vi "publish status.vi"(8 "error in (no error)":errorcluster, 11 "Channel in":refnum<class "SPARC4_Channel.lvclass">) -> (0 "error out":errorcluster, 3 "Channel out":refnum<class "SPARC4_Channel.lvclass">)   [LabVIEW 2018, in "SPARC4_Channel.lvclass"]
uses:
  SPARC4_Channel.lvclass
  State Machine/State Machine.lvclass
  Sim_Ixon_Ultra/Sim_Ixon_Ultra.lvclass
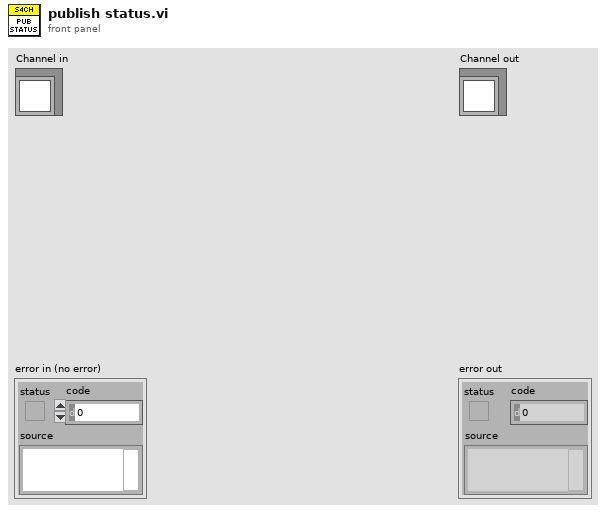
[diagram p1: front panel]
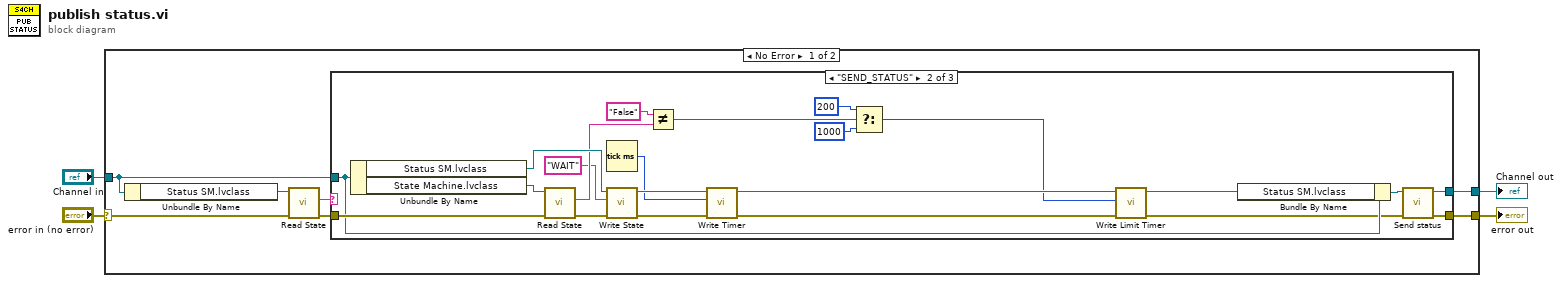
[diagram p0: block diagram]
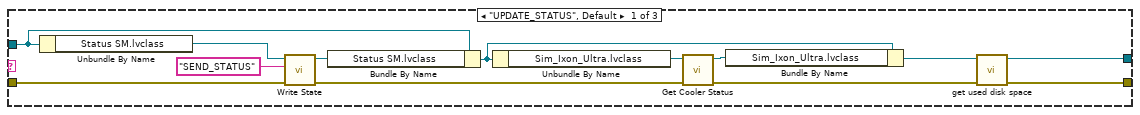
[diagram p2: hidden frame]
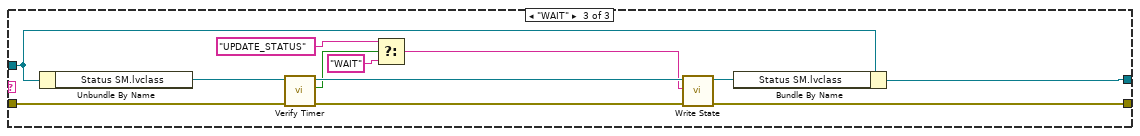
[diagram p3: hidden frame]
diagram:
  n1 = case shown="No Error" "error in (no error)" {
    selector: "error in (no error)" -> [w10 w60]
    tunnel: [w5 w60] -> w3
    tunnel: [w7 w59] -> w1
    tunnel: "Channel in" -> [w6 w59]
    frame No Error {
      n2 = Unbundle By Name(w6) -> ("Status SM.lvclass"=w11:refnum<class "State Machine.lvclass">)
      n3 = call-dynamic "Read State.vi"("error in (no error)"=w10, "State Machine in"=w11) -> ("error out"=w8:errorcluster, "State"=w9:string)  [unwired: 7 in, 1 out]
      n4 = case shown="\"SEND_STATUS\"" w9 {
        tunnel: w6 -> [w19 w30 w57]
        tunnel: w8 -> [w20 w31 w58]
        tunnel: [w14 w26 w51] -> w5
        tunnel: [w12 w25 w55] -> w7
        frame "UPDATE_STATUS", Default {
          n5 = Unbundle By Name(w19) -> ("Status SM.lvclass"=w22:refnum<class "State Machine.lvclass">)
          n6 = call-dynamic "Write State.vi"("error in (no error)"=w20, "State"="SEND_STATUS", "State Machine in"=w22) -> ("error out"=w17:errorcluster, "State Machine out"=w23:refnum<class "State Machine.lvclass">)  [unwired: 7 in]
          n7 = Bundle By Name(cluster=w19, "Status SM.lvclass"=w23) -> (w24:refnum<class "SPARC4_Channel.lvclass">)
          n8 = Unbundle By Name(w24) -> ("Sim_Ixon_Ultra.lvclass"=w18:refnum<class "Sim_Ixon_Ultra.lvclass">)
          n9 = call-dynamic "Get Cooler Status.vi"("error in (no error)"=w17, "CCDCamera in"=w18) -> ("error out"=w15:errorcluster, "CCDCamera out"=w16:refnum<class "Sim_Ixon_Ultra.lvclass">)  [unwired: 8 in]
          n10 = Bundle By Name(cluster=w24, "Sim_Ixon_Ultra.lvclass"=w16) -> (w13:refnum<class "SPARC4_Channel.lvclass">)
          n11 = call "get used disk space.vi"("error in (no error)"=w15, "Channel in"=w13) -> ("error out"=w14:errorcluster, "Channel out"=w12:refnum<class "SPARC4_Channel.lvclass">)  [unwired: 8 in]
        }
        frame "SEND_STATUS" {
          n12 = Unbundle By Name(w30) -> ("Status SM.lvclass"=w39:refnum<class "State Machine.lvclass">, "State Machine.lvclass"=w40:refnum<class "State Machine.lvclass">)
          n13 = call-dynamic "Read State.vi"("error in (no error)"=w31, "State Machine in"=w40) -> ("error out"=w38:errorcluster, "State"=w37:string)  [unwired: 7 in, 1 out]
          n14 = Tick Count (ms)() -> (millisecond timer value=w44:u32)
          n15 = call-dynamic "Write State.vi"("error in (no error)"=w38, "State"="WAIT", "State Machine in"=w39) -> ("error out"=w45:errorcluster, "State Machine out"=w46:refnum<class "State Machine.lvclass">)  [unwired: 7 in]
          n16 = Not Equal?(x="False" ("State"), y=w37) -> (x != y?=w29:bool)
          n17 = call "Write Timer.vi"("error in (no error)"=w45, "Timer"=w44, "State Machine in"=w46) -> ("error out"=w41:errorcluster, "State Machine out"=w43:refnum<class "State Machine.lvclass">)  [unwired: 7 in]
          n18 = Select(t=200, s=w29, f=1000) -> (s? t:f=w36:i32)
          n19 = call "Write Limit Timer.vi"("error in (no error)"=w41, "Limit Timer"=w36, "State Machine in"=w43) -> ("error out"=w27:errorcluster, "State Machine out"=w42:refnum<class "State Machine.lvclass">)  [unwired: 7 in]
          n20 = Bundle By Name(cluster=w30, "Status SM.lvclass"=w42) -> (w28:refnum<class "SPARC4_Channel.lvclass">)
          n21 = call "Send status.vi"("error in (no error)"=w27, "Channel in"=w28) -> ("error out"=w26:errorcluster, "Channel out"=w25:refnum<class "SPARC4_Channel.lvclass">)  [unwired: 8 in]
        }
        frame "WAIT" {
          n22 = Unbundle By Name(w57) -> ("Status SM.lvclass"=w56:refnum<class "State Machine.lvclass">)
          n23 = call "Verify Timer.vi"("error in (no error)"=w58, "State Machine in"=w56) -> ("error out"=w54:errorcluster, "time out"=w47:bool, "State Machine out"=w53:refnum<class "State Machine.lvclass">)  [unwired: 7 in]
          n24 = Select(t="UPDATE_STATUS", s=w47, f="WAIT") -> (s? t:f=w50:string)
          n25 = call-dynamic "Write State.vi"("error in (no error)"=w54, "State"=w50, "State Machine in"=w53) -> ("error out"=w51:errorcluster, "State Machine out"=w52:refnum<class "State Machine.lvclass">)  [unwired: 7 in]
          n26 = Bundle By Name(cluster=w57, "Status SM.lvclass"=w52) -> (w55:refnum<class "SPARC4_Channel.lvclass">)
        }
      }
    }
    frame Error {
    }
  }
  "error out" <- w3
  "Channel out" <- w1
